vi "fillErrors.vi"(8 "error in (no error)":errorcluster, 11 "ElectrometerError in":refnum<class "ElectrometerError.lvclass">) -> (0 "error out":errorcluster, 3 "ElectrometerError out":refnum<class "ElectrometerError.lvclass">)   [LabVIEW 2016, in "ElectrometerError.lvclass"]
uses:
  ElectrometerError.lvclass
  ElectrometerError.lvclass/ElectrometerError.ctl
  Controls/errorType.ctl
  <vilib>/Utility/file.llb/Read Delimited Spreadsheet (string).vi
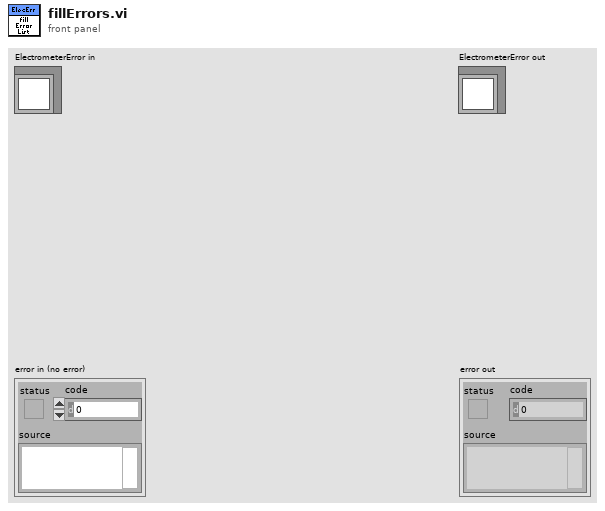
[diagram p1: front panel]
types:
  T1 = typedef "ElectrometerError.lvclass/errorType.ctl" = cluster{"errorType":enum16{"Error", "Warning", "None"}, "errorCode":dbl, "hwError":string, "salError":string}
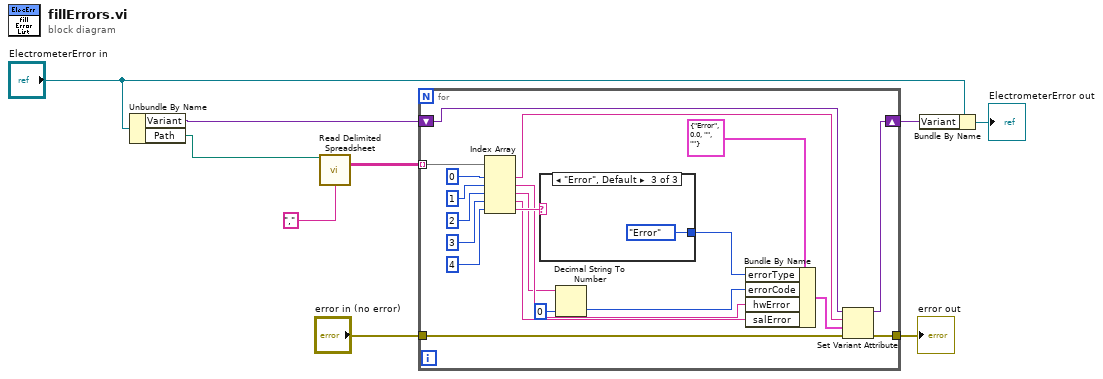
[diagram p0: block diagram]
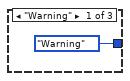
[diagram p2: hidden frame]
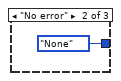
[diagram p3: hidden frame]
diagram:
  n1 = Unbundle By Name("ElectrometerError in") -> ("Variant"=w7:variant, "Path"=w1:path)
  n2 = call-poly <vilib>:"Read Delimited Spreadsheet.vi"("file path (dialog if empty)"=w1, "delimiter (\\t)"="," ("delimiter (\\t)")) -> ("all rows"=w6:string[][])  [unwired: 8 in, 5 out]
  n3 = for {
    tunnel: w6 -> [w29] mode=indexing
    tunnel: "error in (no error)" -> [w22]
    tunnel: [w21] -> w2
    shift-right: [w23] -> w8
    shift-left: w7 -> [w24]
    n4 = Index Array(array=w29, index #1=0 ("index"), index #2=1 ("index"), index #3=2 ("index"), index #4=3 ("index"), index #5=4 ("index")) -> (element #1=w20:string, element #2=w14:string, element #3=w11:string, element #4=w13:string, element #5=w15:string)
    n5 = case shown="\"Error\", Default" w15 {
      tunnel: [enum16{"Error", "Warning", "None"}."Warning" ("errorType") enum16{"Error", "Warning", "None"}."None" ("errorType") enum16{"Error", "Warning", "None"}."Error" ("errorType")] -> w17
      frame "Warning" {
      }
      frame "No error" {
      }
      frame "Error", Default {
      }
    }
    n6 = Decimal String To Number(string=w11, default (0L)=0 ("default (0 I32)")) -> (number=w12:i32)  [unwired: 1 in, 1 out]
    n7 = Bundle By Name(cluster=T1 {"errorType"=enum."Error", "errorCode"=0.0, "hwError"="", "salError"=""} ("error"), "errorType"=w17, "errorCode"=w12, "hwError"=w14, "salError"=w13) -> (w18:T1)
    n8 = Set Variant Attribute(Variant=w24, name=w20, value=w18, error in=w22) -> (Variant out=w23:variant, error out=w21:errorcluster)  [unwired: 1 out]
  }
  "error out" <- w2
  n9 = Bundle By Name(cluster="ElectrometerError in", "Variant"=w8) -> (→"ElectrometerError out":refnum<class "ElectrometerError.lvclass">)
